vi "Export_Data_From_Excel_v1.3_Graph_XY.vi"() -> ()   [LabVIEW 2018]
panel:
  out "XY Graph":cluster{"X":dbl, "Y":dbl}[](graph)
  out "Array 2":dbl[][](array[numeric])
  in  "Open":bool
  in  "Загрузка Excel приложения":refnum<k7>
  in  "Excel._Worksheet 2":refnum<k7>
  in  "Array":string[][](array[string])
  in  "Выбор файла":path
  # "Y"
  # "Z"
  # "№ отм."
  # "X"
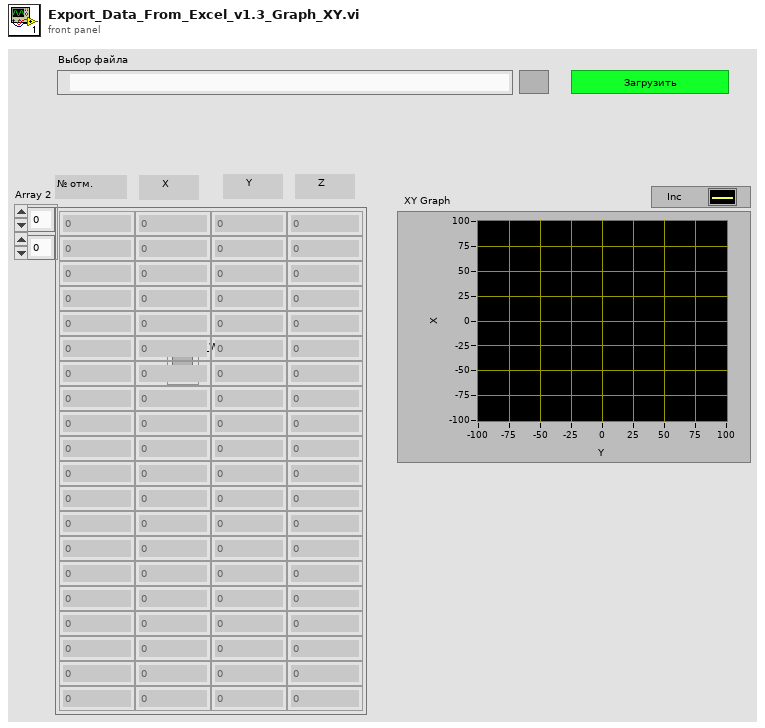
[diagram p1: front panel]
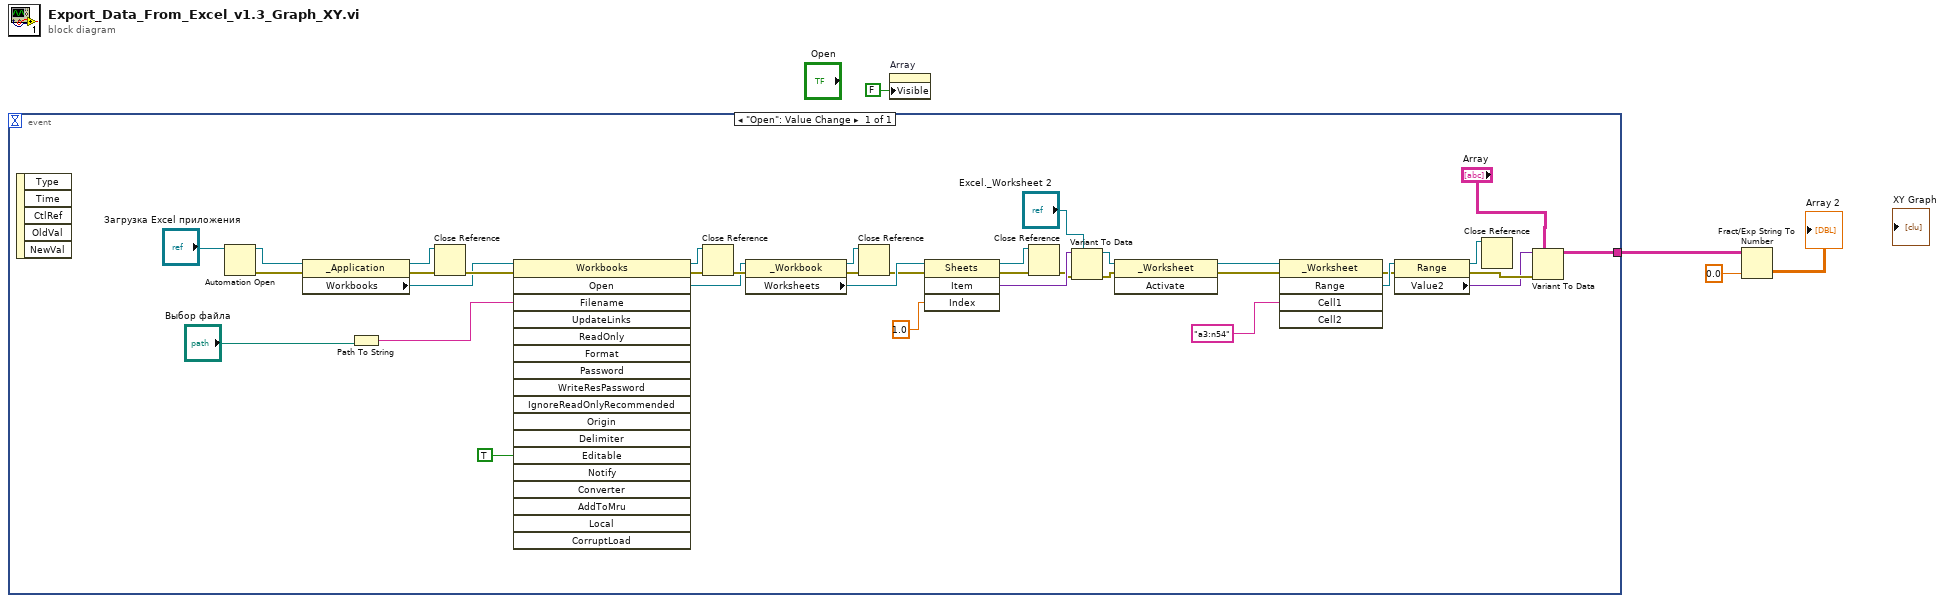
[diagram p0: block diagram]
diagram:
  n1 = event shown="[0] \"Open\": Value Change" {
    selector: _ -> [_]
    dyn-events: _ -> [_]
    timeout: _ -> [_]
    tunnel: [w8] -> w2
    event "Open": Value Change {
      n2 = event-data() -> ()  [unwired: 1 in, 5 out]
      n3 = Automation Open(Automation Refnum="Загрузка Excel приложения") -> (Automation Refnum=w40:refnum<k7>, error out=w28:errorcluster)  [unwired: 3 in]
      n4 = property class="_Application"(reference=w40, error in=w28) -> (reference out=w26:refnum<k7>, error out=w21:errorcluster, "Workbooks"=w11:refnum<k7>)
      n5 = Path To String(path="Выбор файла") -> (string=w9:string)
      n6 = Close Reference(reference=w26, error in (no error)=w21) -> (error out=w20:errorcluster)
      n7 = invoke class="Workbooks" method="Open"(reference=w11, error in=w20, "Filename"=w9, "Editable"=TRUE) -> (reference out=w25:refnum<k7>, error out=w19:errorcluster, "Open"=w10:refnum<k7>)  [unwired: 14 in, 15 out]
      n8 = Close Reference(reference=w25, error in (no error)=w19) -> (error out=w18:errorcluster)
      n9 = property class="_Workbook"(reference=w10, error in=w18) -> (reference out=w24:refnum<k7>, error out=w17:errorcluster, "Worksheets"=w35:refnum<k7>)
      n10 = Close Reference(reference=w24, error in (no error)=w17) -> (error out=w16:errorcluster)
      n11 = invoke class="Sheets" method="Item"(reference=w35, error in=w16, "Index"=1.0) -> (reference out=w23:refnum<k7>, error out=w15:errorcluster, "Item"=w36:variant)  [unwired: 1 in, 1 out]
      n12 = Close Reference(reference=w23, error in (no error)=w15) -> (error out=w14:errorcluster)
      n13 = Variant To Data(error in=w14, type="Excel._Worksheet 2", Variant=w36) -> (data=w38:refnum<k7>, error out=w27:errorcluster)
      n14 = invoke class="_Worksheet" method="Activate"(reference=w38, error in=w27) -> (reference out=w29:refnum<k7>, error out=w13:errorcluster)  [unwired: 1 in, 1 out]
      n15 = invoke class="_Worksheet" method="Range"(reference=w29, error in=w13, "Cell1"="a3:n54") -> (error out=w12:errorcluster, "Range"=w31:refnum<k7>)  [unwired: 2 in, 3 out]
      n16 = property class="Range"(reference=w31, error in=w12) -> (reference out=w22:refnum<k7>, error out=w33:errorcluster, "Value2"=w32:variant)
      n17 = Close Reference(reference=w22) -> ()  [unwired: 1 in, 1 out]
      n18 = Variant To Data(error in=w33, type="Array", Variant=w32) -> (data=w8:string[][])  [unwired: 1 out]
    }
  }
  n19 = property on="Array" class="Arr (strict)"("Visible"=FALSE) -> ()  [unwired: 2 in, 2 out]
  n20 = Fract/Exp String To Number(string=w2, default (0 dbl)=0.0) -> (number=→"Array 2":dbl[][])  [unwired: 2 in, 1 out]
